vi "Flock_Shared_Write Value to Central Process.vi"(8 "error in (no error)":errorcluster, 10 "Message Value":string, 11 "Message Name":string) -> (0 "error out":errorcluster)   [LabVIEW 2013, in "Flock_Shared_Messaging.lvlib" / "Flock_Shared_CentralProcessMessaging.lvlib"]
uses:
  Flock_Shared_CentralProcessMessaging.lvlib
  FGV_Action.ctl
  Flock_Shared_Messaging.lvlib
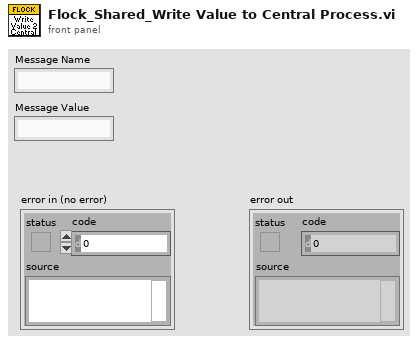
[diagram p1: front panel]
types:
  T1 = typedef "FGV_Action.ctl" = enum16{"Initalize Central", "Initialize Local", "Get", "Delete Local"}
  T2 = typedef "amc_Message Queue.ctl" = refnum<queue>
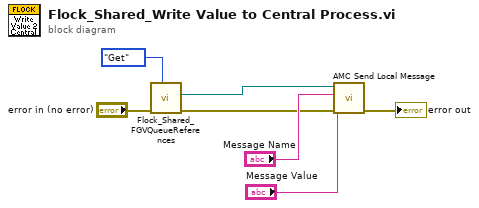
[diagram p0: block diagram]
diagram:
  n1 = call "Flock_Shared_FGVQueueReferences.vi"("Action"=FGV_Action."Get", "error in (no error)"="error in (no error)") -> ("error out"=w3:errorcluster, "Central Queue out"=w4:T2)  [unwired: 7 in, 1 out]
  n2 = call <vilib>:"AMC Send Local Message.vi"("error in (no error)"=w3, "Message Value"="Message Value", "Message Name"="Message Name", "Message Queue in"=w4) -> ("error out"=→"error out":errorcluster)  [unwired: 6 in, 1 out]
